vi "Inizialize map.vi"(11 "Boolean":bool) -> (0 "Map dimesions":dbl[](array[numeric]), 1 "Map initialize":dbl[][](array[numeric]), 2 "Robot start location":dbl[](array[numeric]), 4 "Robot actual location":dbl[](array[numeric]), 5 "Robot angle":dbl)   [LabVIEW 2015]
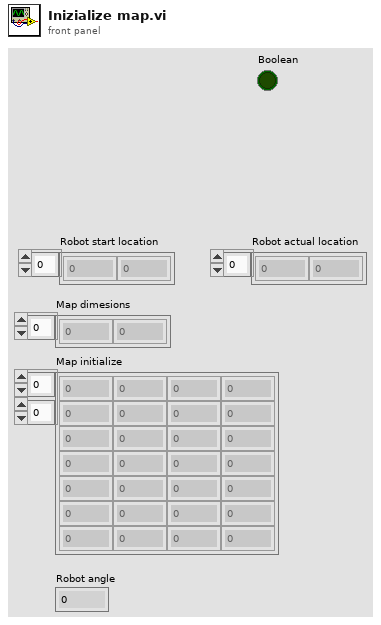
[diagram p1: front panel]
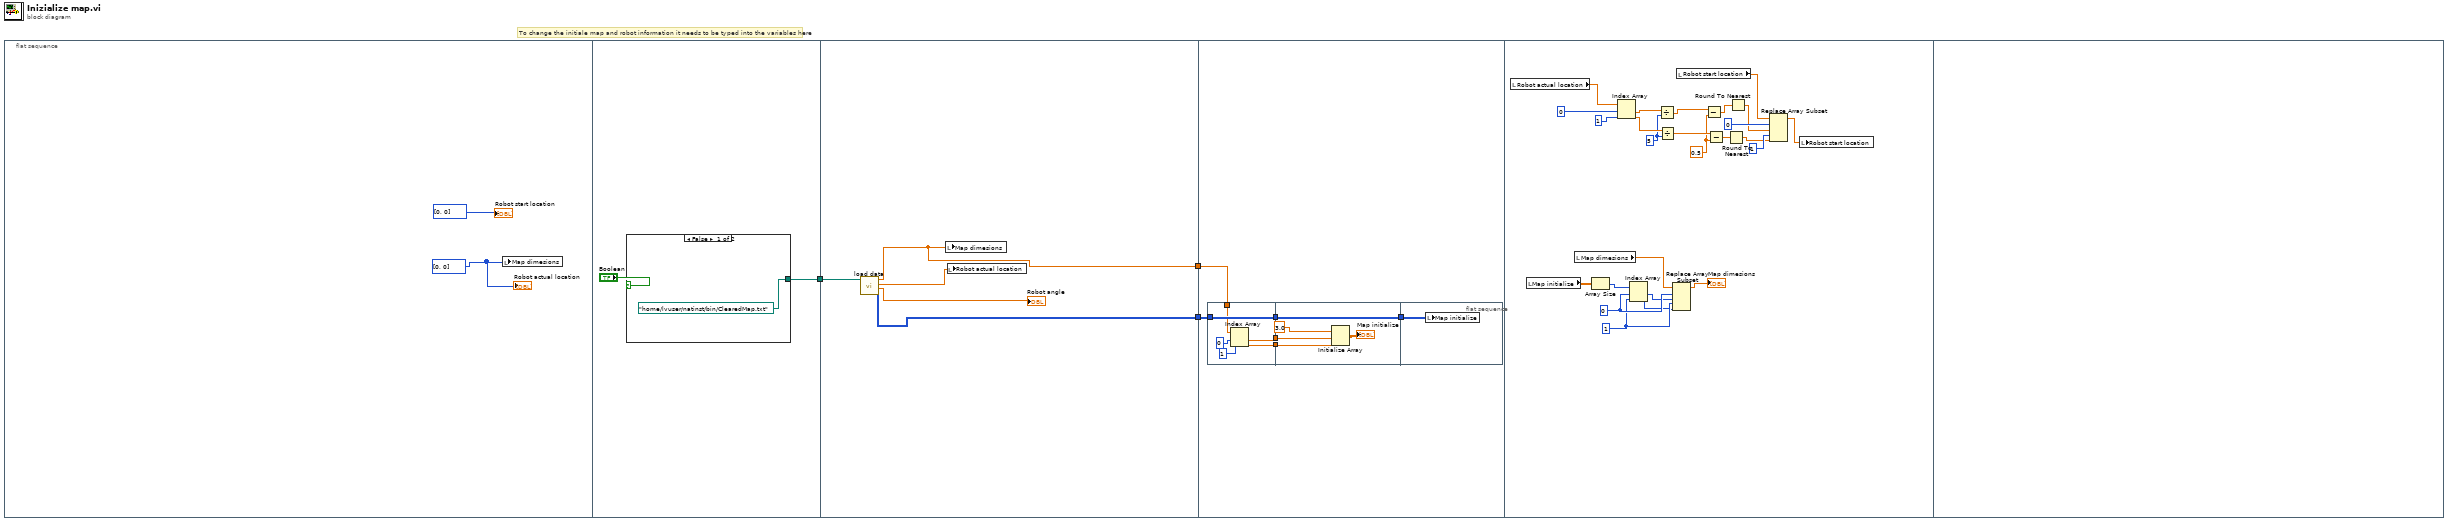
[diagram p0: block diagram]
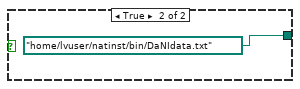
[diagram p2: hidden frame]
diagram:
  # "To change the initiale map and robot information it needs to be typed into the variables here"
  n1 = flat-sequence {
    tunnel: [w6] -> w1
    tunnel: [w13] -> w3
    tunnel: [w12] -> w2
    tunnel: w1 -> [w10]
    tunnel: w3 -> [w18]
    tunnel: w2 -> [w16]
    frame #0 {
      w4 = i32[] [0, 0]
      n2 = local write "Map dimesions"(w4) -> ()
      "Robot start location" <- i32[] [0, 0]
      "Robot actual location" <- w4
    }
    frame #1 {
      n3 = case shown="False" "Boolean" {
        tunnel: [path "/home/lvuser/natinst/bin/ClearedMap.txt" ("file path (use dialog)") path "/home/lvuser/natinst/bin/DaNIdata.txt" ("file path (use dialog)")] -> w6
        frame False {
        }
        frame True {
        }
      }
    }
    frame #2 {
      n4 = call "load data.vi"("file path (use dialog)"=w10) -> ("Obsticle map"=w13:u16[][], "Robot angle"=→"Robot angle":dbl, "Actual robot location"=w14:dbl[], "Map dimensions"=w12:dbl[])  [unwired: 7 in]
      n5 = local write "Map dimesions"(w12) -> ()
      n6 = local write "Robot actual location"(w14) -> ()
    }
    frame #3 {
      n7 = flat-sequence {
        tunnel: w18 -> [w26]
        tunnel: [w26] -> w20
        tunnel: [w25] -> w17
        tunnel: w16 -> [w24]
        tunnel: [w21] -> w15
        tunnel: [w31] -> w19
        tunnel: w20 -> [w31]
        tunnel: w17 -> [w28]
        tunnel: w15 -> [w27]
        tunnel: w19 -> [w32]
        frame #0 {
          n8 = Index Array(array=w24, index #1=0, index #2=1) -> (element #1=w25:dbl, element #2=w21:dbl)
        }
        frame #1 {
          n9 = Initialize Array(3.0, w28, w27) -> (→"Map initialize":dbl[][])
        }
        frame #2 {
          n10 = local write "Map initialize"(w32) -> ()
        }
      }
    }
    frame #4 {
      w37 = 0.5
      w44 = 5
      w54 = 1
      w55 = 0
      n11 = local read "Robot actual location"() -> (w49:dbl[])
      n12 = local read "Map initialize"() -> (w57:dbl[][])
      n13 = local read "Map dimesions"() -> (w50:dbl[])
      n14 = Array Size(array=w57) -> (size(s)=w56:i32[])
      n15 = Index Array(array=w49, index #1=0, index #2=1) -> (element #1=w46:dbl, element #2=w45:dbl)
      n16 = Index Array(array=w56, index #1=w55, index #2=w54) -> (element #1=w53:i32, element #2=w52:i32)
      n17 = Divide(x=w46, y=w44) -> (x/y=w42:dbl)
      n18 = Divide(x=w45, y=w44) -> (x/y=w43:dbl)
      n19 = Replace Array Subset(array=w50, new element #1=w53, index #1=w55, new element #2=w52, index #2=w54) -> (→"Map dimesions":dbl[])
      n20 = local read "Robot start location"() -> (w41:dbl[])
      n21 = Subtract(x=w42, y=w37) -> (x-y=w34:dbl)
      n22 = Subtract(x=w43, y=w37) -> (x-y=w36:dbl)
      n23 = Round To Nearest(number=w36) -> (nearest integer value=w35:dbl)
      n24 = Round To Nearest(number=w34) -> (nearest integer value=w33:dbl)
      n25 = Replace Array Subset(array=w41, new element #1=w33, index #1=0, new element #2=w35, index #2=1) -> (w40:dbl[])
      n26 = local write "Robot start location"(w40) -> ()
    }
    frame #5 {
    }
  }
